vi "Add Report Section.vi"(6 "Step Number":i32, 7 "Report Path":path, 8 "error in (no error)":errorcluster, 9 "Report Data":T1, 10 "Report in":refnum<class "NI_report.lvclass">, 11 "Boolean Assertion in":refnum<class "Boolean Assertion.lvclass">) -> (0 "error out":errorcluster, 2 "Report out":refnum<class "NI_report.lvclass">, 3 "Boolean Assertion out":refnum<class "Boolean Assertion.lvclass">)   [LabVIEW 2020, in "MacroAssert.lvlib" / "Boolean Assertion.lvclass"]
uses:
  Boolean Assertion.lvclass
  Boolean Assertion.lvclass/Boolean Assertion.ctl
  <vilib>/Utility/NIReport.llb/NI_report.lvclass
  C:/Users/acasalen/Documents/LabVIEW Data/Projects/MacroAssert/source/Classes/Assertion Step/Assertion Step.lvclass
  C:/Users/acasalen/Documents/LabVIEW Data/Projects/MacroAssert/source/Classes/Step/Step.lvclass
  C:/Users/acasalen/Documents/LabVIEW Data/Projects/MacroAssert/source/Classes/Boolean Assertion/Boolean Assertion.lvclass
  Assertion Step/Assertion Step.lvclass
  CTLs/Report Data.ctl
  MacroAssert.lvlib
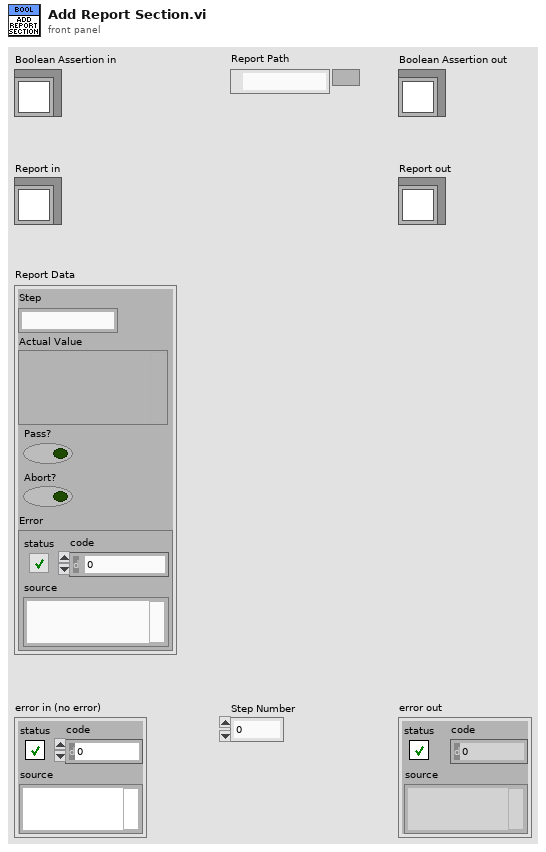
[diagram p1: front panel]
types:
  T1 = typedef "MacroAssert.lvlib/Report Data.ctl" = cluster{"Step":string, "Actual Value":variant, "Pass?":bool, "Abort?":bool, "Error":errorcluster}
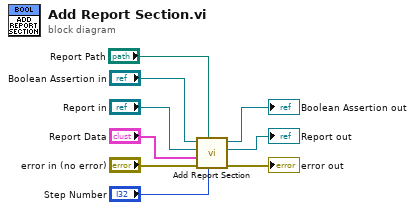
[diagram p0: block diagram]
diagram:
  n1 = call-parent "Add Report Section.vi"("Step Number"="Step Number", "Report Path"="Report Path", "error in (no error)"="error in (no error)", "Report Data"="Report Data", "Report in"="Report in", "Step in"="Boolean Assertion in") -> ("error out"=→"error out":errorcluster, "Report out"=→"Report out":refnum<class "NI_report.lvclass">, "Step out"=→"Boolean Assertion out":refnum<class "Boolean Assertion.lvclass">)  [unwired: 3 in]
